vi "Untitled 3.vi"() -> ()   [LabVIEW 2014]
panel:
  out "Array 5":dbl[](array[numeric])
  out "Numeric 5":dbl
  in  "Numeric 4":dbl
  in  "Numeric 3":dbl
  out "Array 4":void[](array[numeric])
  in  "Numeric 2":dbl
  out "Numeric":dbl
  out "Array 3":dbl[](array[numeric])
  out "Array 2":dbl[](array[numeric])
  out "Array":dbl[](array[numeric])
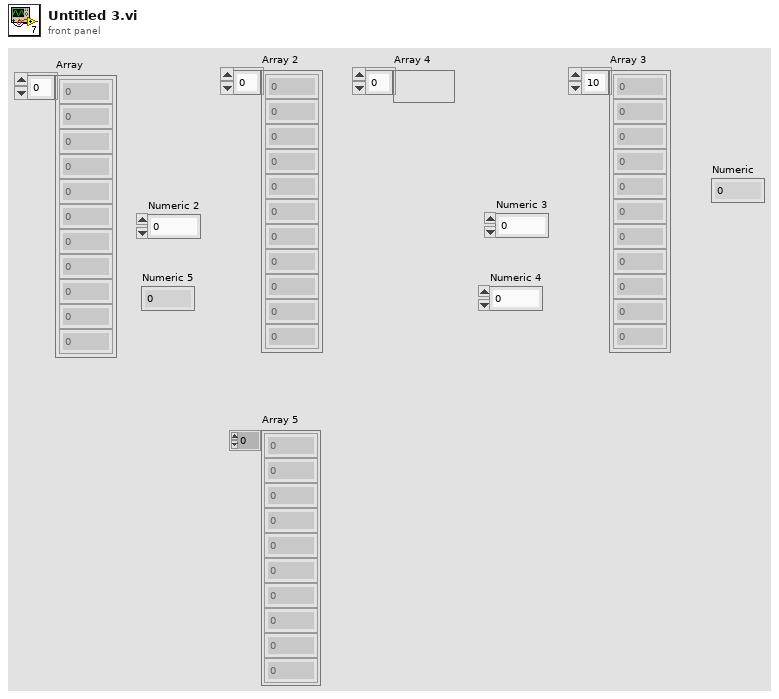
[diagram p1: front panel]
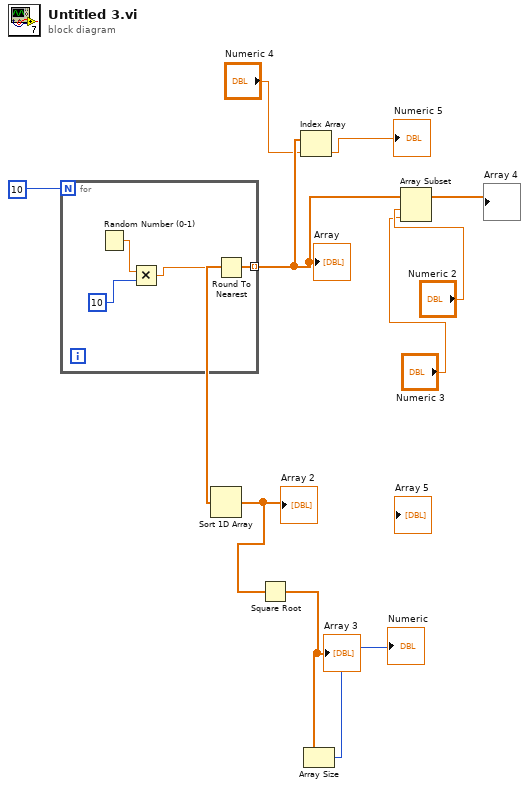
[diagram p0: block diagram]
diagram:
  n1 = for {
    N: 10 -> [_]
    tunnel: [w11] -> w3 mode=indexing
    n2 = Random Number (0-1)() -> (number: 0 to 1=w14:dbl)
    n3 = Multiply(x=w14, y=10) -> (x*y=w12:dbl)
    n4 = Round To Nearest(number=w12) -> (nearest integer value=w11:dbl)
  }
  "Array" <- w3
  n5 = Sort 1D Array(array=w3) -> (sorted array=w9:dbl[])
  "Array 2" <- w9
  n6 = Square Root(x=w9) -> (sqrt(x)=w8:dbl[])
  "Array 3" <- w8
  n7 = Index Array(array=w3, index="Numeric 4") -> (element=→"Numeric 5":dbl)
  n8 = Array Size(array=w8) -> (size(s)=→"Numeric":i32)
  n9 = Array Subset(array=w3, index="Numeric 2", length="Numeric 3") -> (→"Array 4":dbl[])
